vi "Close.vi"(8 "error in (no error)":errorcluster, 11 "NI DMM in":refnum<class "NI DMM.lvclass">) -> (0 "error out":errorcluster, 3 "NI DMM out":refnum<class "NI DMM.lvclass">)   [LabVIEW 2020, in "NI DMM.lvclass"]
uses:
  NI DMM.lvclass
  NI DMM.lvclass/NI DMM.ctl
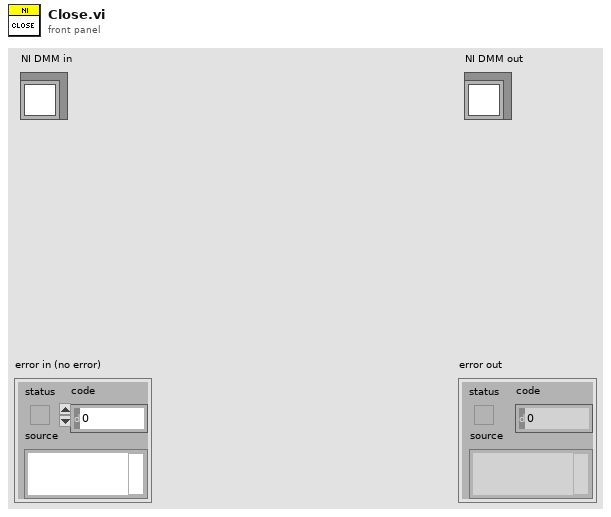
[diagram p1: front panel]
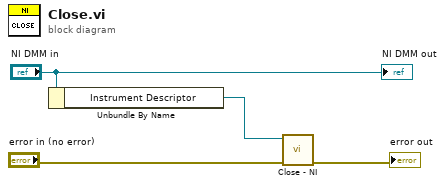
[diagram p0: block diagram]
diagram:
  n1 = Unbundle By Name("NI DMM in") -> ("Instrument Descriptor"=w3:refnum<k15>)
  n2 = call "Close - NI.vi"("error in (no error)"="error in (no error)", "instrument handle"=w3) -> ("error out"=→"error out":errorcluster)  [unwired: 9 in]
  "NI DMM out" <- "NI DMM in"
